vi "lightsource-wl-set.vi"(0 "NKT Input Control":T2={"Emission"=FALSE, "Operation Mode"=FALSE, "Power Level"=5.0, "Feedback Level"=0.0, "Short Wavelength (nm)"=560.0, "Long Wavelength (nm)"=580.0, "UV Wavelength (nm)"=400.0} caption="NKT Input" {"UV Wavelength (nm)" min=350.0 max=480.0 step=1.0 format="%.1f"; "Long Wavelength (nm)" min=400.0 max=850.0 step=1.0 format="%.1f"; "Short Wavelength (nm)" min=400.0 max=850.0 step=1.0 format="%.1f"; "Feedback Level" min=0.0 max=90.0 step=0.1 format="%.1f%%"; "Power Level" min=5.0 max=100.0 step=0.1 format="%.1f%%"}, 1 "Select NKT System":enum32{"SuperK Varia (VIS)", "Extend-UV"}(radio), 2 "Wavelength Cluster":T3 {"Long Wavelength (nm)" format="%.1f"; "Short Wavelength (nm)" format="%.1f"}, 3 "NKT Output Control":T1 caption="NKT Output" {"UV Wavelength (nm)" format="%.1f"; "Long Wavelength (nm)" format="%.1f"; "Short Wavelength (nm)" format="%.1f"; "Feedback Level" format="%.1f%%"; "Power Level" format="%.1f%%"; "Temp (°C)" format="%.1f"}, 4 "VISA in":refnum<visa-resource-name>, 6 "First Loop?":bool=TRUE) -> (5 "NKT Input Indicator":T2={"Emission"=FALSE, "Operation Mode"=FALSE, "Power Level"=5.0, "Feedback Level"=0.0, "Short Wavelength (nm)"=560.0, "Long Wavelength (nm)"=580.0, "UV Wavelength (nm)"=400.0} caption="NKT Input" {"UV Wavelength (nm)" min=350.0 max=480.0 step=1.0 format="%.1f"; "Long Wavelength (nm)" min=400.0 max=850.0 step=1.0 format="%.1f"; "Short Wavelength (nm)" min=400.0 max=850.0 step=1.0 format="%.1f"; "Feedback Level" min=0.0 max=90.0 step=0.1 format="%.1f%%"; "Power Level" min=5.0 max=100.0 step=0.1 format="%.1f%%"}, 7 "NKT Output Indicator":T1 caption="NKT Output" {"UV Wavelength (nm)" format="%.1f"; "Long Wavelength (nm)" format="%.1f"; "Short Wavelength (nm)" format="%.1f"; "Feedback Level" format="%.1f%%"; "Power Level" format="%.1f%%"; "Temp (°C)" format="%.1f"})   [LabVIEW 2015]
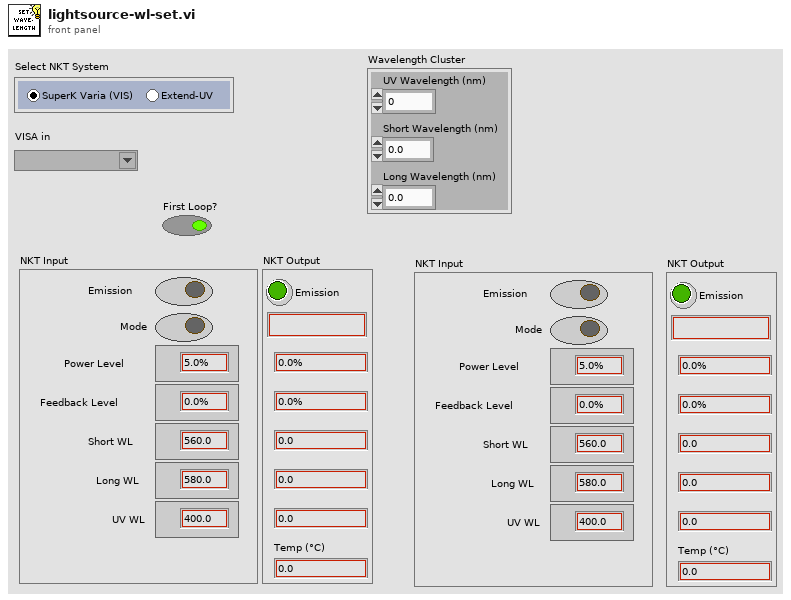
[diagram p1: front panel]
types:
  T1 = cluster{"Emission":bool, "Operation Mode":string, "Power Level":dbl, "Feedback Level":dbl, "Short Wavelength (nm)":dbl, "Long Wavelength (nm)":dbl, "UV Wavelength (nm)":dbl, "Temp (°C)":dbl}
  T2 = cluster{"Emission":bool, "Operation Mode":bool, "Power Level":dbl, "Feedback Level":dbl, "Short Wavelength (nm)":dbl, "Long Wavelength (nm)":dbl, "UV Wavelength (nm)":dbl}
  T3 = cluster{"UV Wavelength (nm)":dbl, "Short Wavelength (nm)":dbl, "Long Wavelength (nm)":dbl}
  T4 = cluster{"UV Wavelength (nm)":i32, "Short Wavelength (nm)":i32, "Long Wavelength (nm)":i32}
  T5 = cluster{"Destination":u8, "Source":u8, "Register":u8, "Array":i16[], "WriteNotRead":bool, "ReadWithPreample":bool, "Ring":u16, "String":string, "Long":i32}
  T6 = cluster{"OpenPort":bool, "ClosePort":bool, "Baudrate":i32, "Wait":u16, "ReadWrite":bool}
  T7 = cluster{"Source":u8, "TelegramType":u8, "Register":u8, "Destination":u8, "TelegramReceived":bool, "CRC error":bool, "PayloadByteArray":u8[], "(hi.lo)":u16, "Crc16":u16, "Long":i32, "PayloadIntArray":u16[], "String":string}
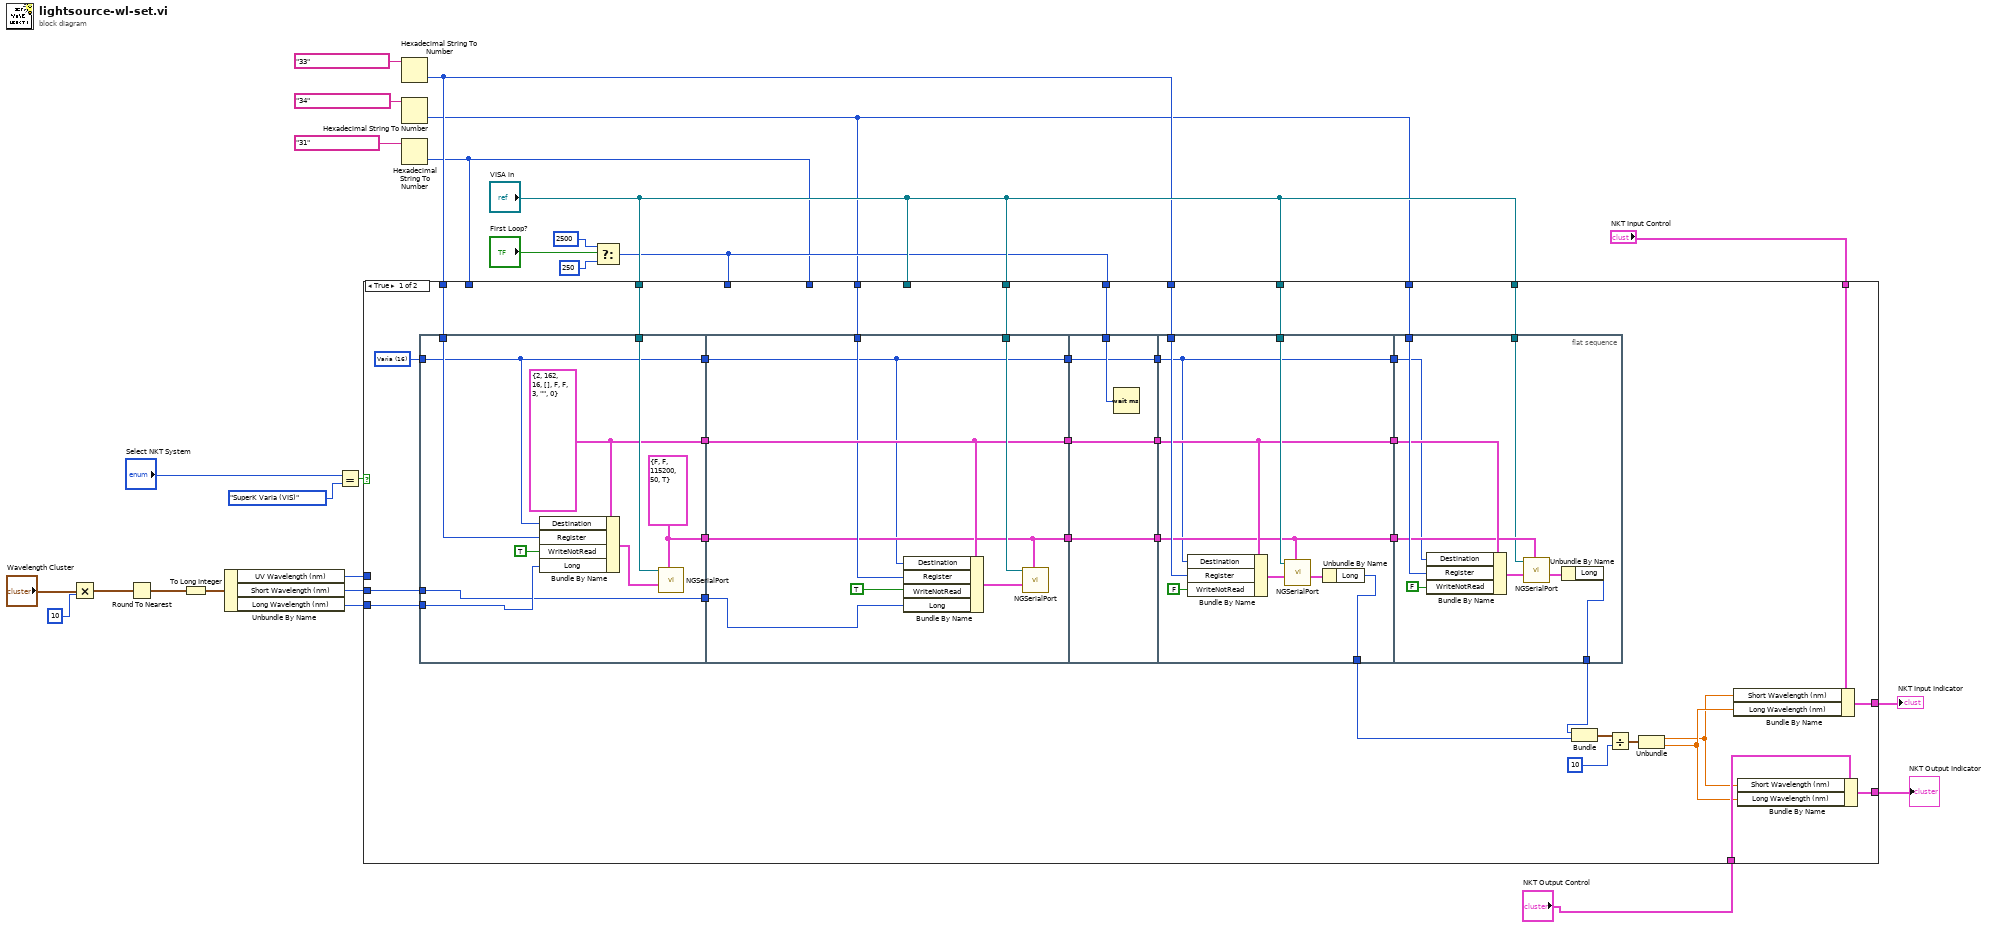
[diagram p0: block diagram]
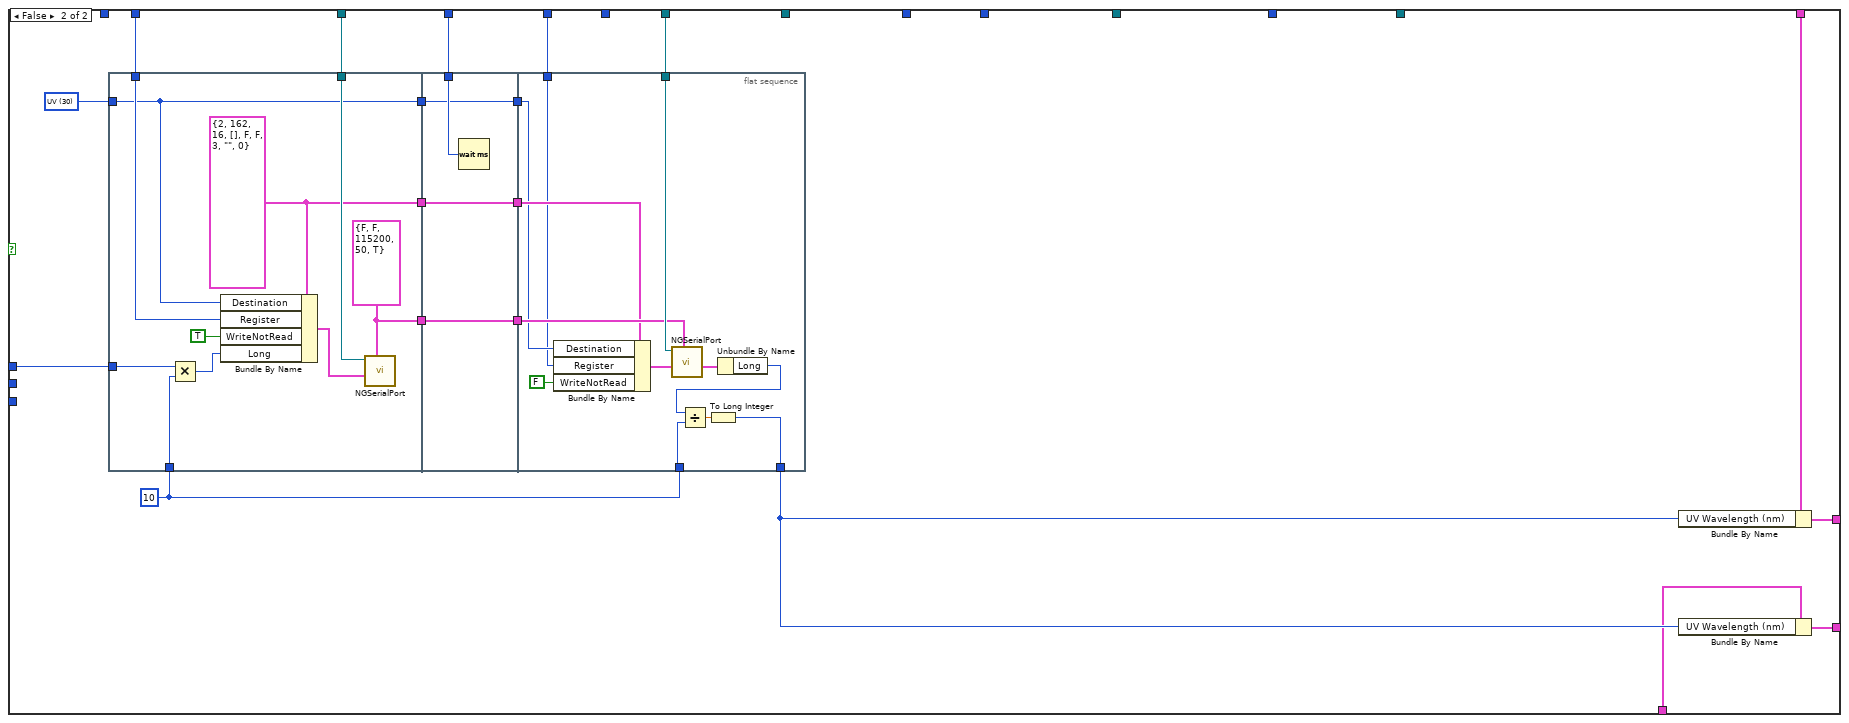
[diagram p2: hidden frame]
diagram:
  n1 = Multiply(x="Wavelength Cluster", y=10) -> (x*y=w4:T3)
  n2 = Round To Nearest(number=w4) -> (nearest integer value=w3:T3)
  n3 = To Long Integer(number=w3) -> (32bit integer=w2:T4)
  n4 = Unbundle By Name(w2) -> ("UV Wavelength (nm)"=w19:i32, "Short Wavelength (nm)"=w1:i32, "Long Wavelength (nm)"=w20:i32)
  n5 = Equal?(x="Select NKT System", y=enum32{"SuperK Varia (VIS)", "Extend-UV"}."SuperK Varia (VIS)" ("Select NKT System")) -> (x = y?=w18:bool)
  n6 = Hexadecimal String To Number(string="33" ("Varia Register 13")) -> (number=w15:u32)  [unwired: 2 in, 1 out]
  n7 = Hexadecimal String To Number(string="34" ("Varia Register 13")) -> (number=w14:u32)  [unwired: 2 in, 1 out]
  n8 = Hexadecimal String To Number(string="31" ("Varia Register 13")) -> (number=w11:u32)  [unwired: 2 in, 1 out]
  n9 = Select(t=u32 2500 ("milliseconds to wait"), s="First Loop?", f=u32 250) -> (s? t:f=w16:u32)
  n10 = case shown="True" w18 {
    tunnel: w15 -> [w54 _]
    tunnel: w14 -> [w53 _]
    tunnel: "VISA in" -> [w52 w116]
    tunnel: [w51 w114] -> w10
    tunnel: [w50 w110] -> w7
    tunnel: w20 -> [w49 _]
    tunnel: w19 -> [_ w112]
    tunnel: "NKT Input Control" -> [w48 w111]
    tunnel: "NKT Output Control" -> [w47 w109]
    tunnel: "VISA in" -> [w46 _]
    tunnel: "VISA in" -> [w45 _]
    tunnel: "VISA in" -> [w44 _]
    tunnel: "VISA in" -> [_ w108]
    tunnel: w16 -> [w43 _]
    tunnel: w16 -> [_ w107]
    tunnel: w15 -> [w42 _]
    tunnel: w14 -> [w41 _]
    tunnel: w11 -> [_ w103]
    tunnel: w11 -> [_ w102]
    tunnel: w1 -> [w34 _]
    frame True {
      w40 = u16 16 items=["SuperK"=15, "Varia"=16, "UV"=30] ("Module 9")
      n11 = flat-sequence {
        tunnel: w52 -> [w69]
        tunnel: [w68] -> w61
        tunnel: [w67] -> w62
        tunnel: w42 -> [w66]
        tunnel: w49 -> [w64]
        tunnel: w40 -> [w65]
        tunnel: [w65] -> w38
        tunnel: [w63] -> w35
        tunnel: w34 -> [w63]
        tunnel: w46 -> [w77]
        tunnel: [w76] -> w60
        tunnel: w53 -> [w75]
        tunnel: [w74] -> w59
        tunnel: w62 -> [w74]
        tunnel: w61 -> [w76]
        tunnel: [w73] -> w39
        tunnel: w38 -> [w73]
        tunnel: w35 -> [w72]
        tunnel: w60 -> [w83]
        tunnel: [w83] -> w58
        tunnel: w59 -> [w82]
        tunnel: [w82] -> w57
        tunnel: w43 -> [w81]
        tunnel: w39 -> [w80]
        tunnel: [w80] -> w37
        tunnel: w58 -> [w87]
        tunnel: w54 -> [w90]
        tunnel: w45 -> [w89]
        tunnel: w57 -> [w86]
        tunnel: [w87] -> w56
        tunnel: [w86] -> w55
        tunnel: w37 -> [w85]
        tunnel: [w85] -> w36
        tunnel: [w84] -> w33
        tunnel: w41 -> [w99]
        tunnel: w56 -> [w98]
        tunnel: w55 -> [w97]
        tunnel: w44 -> [w96]
        tunnel: w36 -> [w94]
        tunnel: [w93] -> w32
        frame #0 {
          w68 = T5 {"Destination"=2, "Source"=162, "Register"=16, "Array"=[], "WriteNotRead"=FALSE, "ReadWithPreample"=FALSE, "Ring"=3, "String"="", "Long"=0} ("InParameters")
          w67 = T6 {"OpenPort"=FALSE, "ClosePort"=FALSE, "Baudrate"=115200, "Wait"=50, "ReadWrite"=TRUE} ("PortParameters")
          n12 = Bundle By Name(cluster=w68, "Destination"=w65, "Register"=w66, "WriteNotRead"=TRUE, "Long"=w64) -> (w70:T5)
          n13 = call "NGSerialPort.vi"("PortParameters"=w67, "InParameters"=w70, "VISA in"=w69) -> ()  [unwired: 6 in, 3 out]
        }
        frame #1 {
          n14 = Bundle By Name(cluster=w76, "Destination"=w73, "Register"=w75, "WriteNotRead"=TRUE, "Long"=w72) -> (w79:T5)
          n15 = call "NGSerialPort.vi"("PortParameters"=w74, "InParameters"=w79, "VISA in"=w77) -> ()  [unwired: 6 in, 3 out]
        }
        frame #2 {
          n16 = Wait (ms)(milliseconds to wait=w81) -> ()  [unwired: 1 out]
        }
        frame #3 {
          n17 = Bundle By Name(cluster=w87, "Destination"=w85, "Register"=w90, "WriteNotRead"=FALSE) -> (w92:T5)
          n18 = call "NGSerialPort.vi"("PortParameters"=w86, "InParameters"=w92, "VISA in"=w89) -> ("OutParameters"=w88:T7)  [unwired: 6 in, 2 out]
          n19 = Unbundle By Name(w88) -> ("Long"=w84:i32)
        }
        frame #4 {
          n20 = Bundle By Name(cluster=w98, "Destination"=w94, "Register"=w99, "WriteNotRead"=FALSE) -> (w95:T5)
          n21 = call "NGSerialPort.vi"("PortParameters"=w97, "InParameters"=w95, "VISA in"=w96) -> ("OutParameters"=w101:T7)  [unwired: 6 in, 2 out]
          n22 = Unbundle By Name(w101) -> ("Long"=w93:i32)
        }
      }
      n23 = Bundle("Long"=w32, "Long"=w33) -> (w31:cluster{"Long":i32, "Long":i32})  [unwired: 1 in]
      n24 = Divide(x=w31, y=10) -> (x/y=w29:cluster{"Long":dbl, "Long":dbl})
      n25 = Unbundle(w29) -> ("Long"=w27:dbl, "Long"=w28:dbl)
      n26 = Bundle By Name(cluster=w48, "Short Wavelength (nm)"=w27, "Long Wavelength (nm)"=w28) -> (w51:T2)
      n27 = Bundle By Name(cluster=w47, "Short Wavelength (nm)"=w27, "Long Wavelength (nm)"=w28) -> (w50:T1)
    }
    frame False {
      w113 = 10 ("y")
      w105 = u16 30 items=["SuperK"=15, "Varia"=16, "UV"=30] ("Module 9")
      n28 = flat-sequence {
        tunnel: w116 -> [w128]
        tunnel: [w127] -> w119
        tunnel: [w126] -> w120
        tunnel: w113 -> [w124]
        tunnel: w112 -> [w123]
        tunnel: [w121] -> w106
        tunnel: w105 -> [w121]
        tunnel: w103 -> [w122]
        tunnel: [w134] -> w118
        tunnel: [w133] -> w117
        tunnel: w107 -> [w132]
        tunnel: w119 -> [w134]
        tunnel: w120 -> [w133]
        tunnel: w106 -> [w131]
        tunnel: [w131] -> w104
        tunnel: w118 -> [w137]
        tunnel: w108 -> [w144]
        tunnel: w117 -> [w142]
        tunnel: [w139] -> w115
        tunnel: w113 -> [w140]
        tunnel: w104 -> [w136]
        tunnel: w102 -> [w135]
        frame #0 {
          w127 = T5 {"Destination"=2, "Source"=162, "Register"=16, "Array"=[], "WriteNotRead"=FALSE, "ReadWithPreample"=FALSE, "Ring"=3, "String"="", "Long"=0} ("InParameters")
          w126 = T6 {"OpenPort"=FALSE, "ClosePort"=FALSE, "Baudrate"=115200, "Wait"=50, "ReadWrite"=TRUE} ("PortParameters")
          n29 = Multiply(x=w123, y=w124) -> (x*y=w125:i32)
          n30 = Bundle By Name(cluster=w127, "Destination"=w121, "Register"=w122, "WriteNotRead"=TRUE, "Long"=w125) -> (w129:T5)
          n31 = call "NGSerialPort.vi"("PortParameters"=w126, "InParameters"=w129, "VISA in"=w128) -> ()  [unwired: 6 in, 3 out]
        }
        frame #1 {
          n32 = Wait (ms)(milliseconds to wait=w132) -> ()  [unwired: 1 out]
        }
        frame #2 {
          n33 = Bundle By Name(cluster=w137, "Destination"=w136, "Register"=w135, "WriteNotRead"=FALSE) -> (w146:T5)
          n34 = call "NGSerialPort.vi"("PortParameters"=w142, "InParameters"=w146, "VISA in"=w144) -> ("OutParameters"=w143:T7)  [unwired: 6 in, 2 out]
          n35 = Unbundle By Name(w143) -> ("Long"=w141:i32)
          n36 = Divide(x=w141, y=w140) -> (x/y=w138:dbl)
          n37 = To Long Integer(number=w138) -> (32bit integer=w139:i32)
        }
      }
      n38 = Bundle By Name(cluster=w111, "UV Wavelength (nm)"=w115) -> (w114:T2)
      n39 = Bundle By Name(cluster=w109, "UV Wavelength (nm)"=w115) -> (w110:T1)
    }
  }
  "NKT Input Indicator" <- w10
  "NKT Output Indicator" <- w7
